vi "Path of Caller.vi"() -> (0 "VI Name":string, 1 "Full VI Path":path, 2 "VI Directory":path)   [LabVIEW 2017, in "Drivers.lvlib" / "ASI TG-1000.lvlib"]
uses:
  ASI TG-1000.lvlib
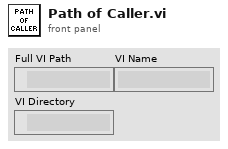
[diagram p1: front panel]
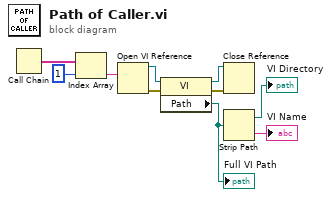
[diagram p0: block diagram]
diagram:
  n1 = Call Chain() -> (call chain=w10:string[])
  n2 = Index Array(array=w10, index=1) -> (element=w8:string)
  n3 = Open VI Reference(vi path=w8) -> (vi reference=w7:refnum<vi>, error out=w6:errorcluster)  [unwired: 5 in]
  n4 = property class="VI"(reference=w7, error in=w6) -> (reference out=w5:refnum<vi>, error out=w4:errorcluster, "Path"=w3:path)
  "Full VI Path" <- w3
  n5 = Close Reference(reference=w5, error in (no error)=w4) -> ()  [unwired: 1 out]
  n6 = Strip Path(path=w3) -> (stripped path=→"VI Directory":path, name=→"VI Name":string)
